vi "State Process.vi"(8 "error in (no error)":errorcluster, 11 "View Model":T1) -> (0 "error out":errorcluster, 3 "View Model":T1)   [LabVIEW 2013]
doc: "Performs actions specific to a state."
uses:
  View Model/Controls/View Model.ctl
  Error/Controls/Error Model.ctl
  Error/Controls/Error Types.ctl
  View Model/Controls/Shared Model.ctl
  Controls/Elevator Model.ctl
  Controls/Controller Overhead.ctl
  Controls/Elevator States.ctl
  Controls/Elevator Location.ctl
  Controls/Elevator Command Event.ctl
  Controls/Elevator Commands.ctl
  Configuration/Controls/Configuration Model.ctl
  Configuration/Controls/Configuration Data.ctl
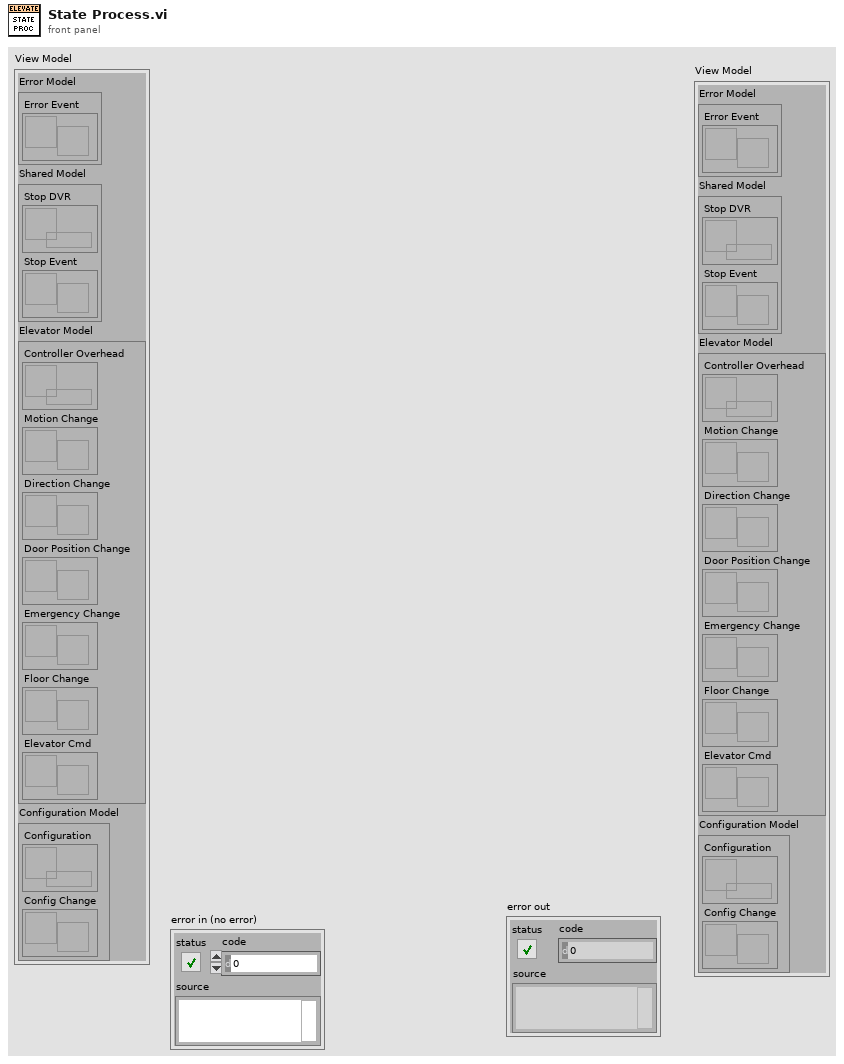
[diagram p1: front panel]
types:
  T1 = typedef "View Model.ctl" = cluster{"Error Model":T2, "Shared Model":T3, "Elevator Model":T4, "Configuration Model":T5}
  T2 = typedef "Error Model.ctl" = cluster{"Error Event":refnum<user-event>}
  T3 = typedef "Shared Model.ctl" = cluster{"Stop DVR":refnum<data-value>, "Stop Event":refnum<user-event>}
  T4 = typedef "Elevator Model.ctl" = cluster{"Controller Overhead":refnum<data-value>, "Motion Change":refnum<user-event>, "Direction Change":refnum<user-event>, "Door Position Change":refnum<user-event>, "Emergency Change":refnum<user-event>, "Floor Change":refnum<user-event>, "Elevator Cmd":refnum<user-event>}
  T5 = typedef "Configuration Model.ctl" = cluster{"Configuration":refnum<data-value>, "Config Change":refnum<user-event>}
  T6 = typedef "Elevator States.ctl" = enum16{"Initial State", "Open Doors", "Close Doors", "Start Move", "Move", "Finish Move", "Emergency", "Analysis"}
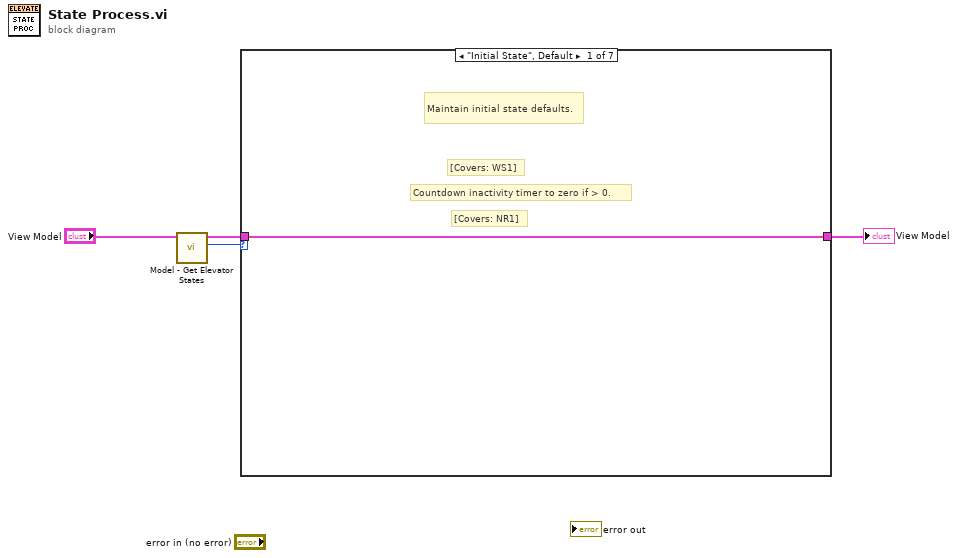
[diagram p0: block diagram]
diagram:
  n1 = call "Model - Get Elevator States.vi"("View Model"="View Model") -> ("Elevator State"=w3:T6, "View Model"=w2:T1)  [unwired: 7 in, 2 out]
  n2 = case shown="\"Initial State\", Default" w3 {
    tunnel: w2 -> [w5 w6 w7 w8 w9 w10 w11]
    tunnel: [w5 w6 w7 w8 w9 w10 w11] -> w1
    frame "Initial State", Default {
      # "[Covers: NR1]"
      # "Countdown inactivity timer to zero if > 0."
      # "[Covers: WS1]"
      # "Maintain initial state defaults."
    }
    frame "Open Doors" {
      # "[Covers: SS1]"
      # "Send digital output to open doors. Fire door open event."
    }
    frame "Close Doors" {
    }
    frame "Start Move" {
    }
    frame "Emergency" {
    }
    frame "Move" {
      # "[Covers: CT1A]"
      # "[Covers: SS4A]"
      # "Update elapsed time and elevator location."
    }
    frame "Finish Move" {
    }
  }
  "View Model" <- w1
